vi "timetest2.vi"() -> ()   [LabVIEW 2015]
uses:
  BERTTA.dll
panel:
  in  "direction":i32
  out "return type 2":dbl
  in  "rt":i32
  in  "Tcurrent":dbl
  in  "Tset":dbl
  in  "enable":i32
  out "return type":i32
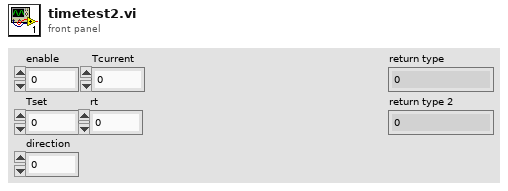
[diagram p1: front panel]
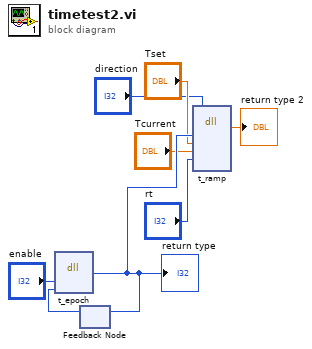
[diagram p0: block diagram]
diagram:
  n1 = feedback #1() -> (w8:i32)  [unwired: 1 in]
  n2 = dll-call lib="C:/Users/xlaraser/Documents/Visual Studio 2017/Projects/Bertta/BERTTA/Debug/BERTTA.dll" fn="t_epoch"("enable"="enable", "start_time"=w8) -> ("return type"=w6:i32)  [unwired: 5 in, 2 out]
  "return type" <- w6
  n3 = feedback-in #1(w6) -> ()
  n4 = dll-call lib="C:/Users/xlaraser/Documents/Visual Studio 2017/Projects/Bertta/BERTTA/Debug/BERTTA.dll" fn="t_ramp"("start_time"=w6, "Tset"="Tset", "Tcurrent"="Tcurrent", "rt"="rt", "direction"="direction") -> ("return type"=→"return type 2":dbl)  [unwired: 8 in, 2 out]
